vi "SetExtSignalPol.vi"(8 "错误输入（无错误）":errorcluster, 10 "外同步信号极性":u8) -> (0 "错误输出":errorcluster)   [LabVIEW 2018]
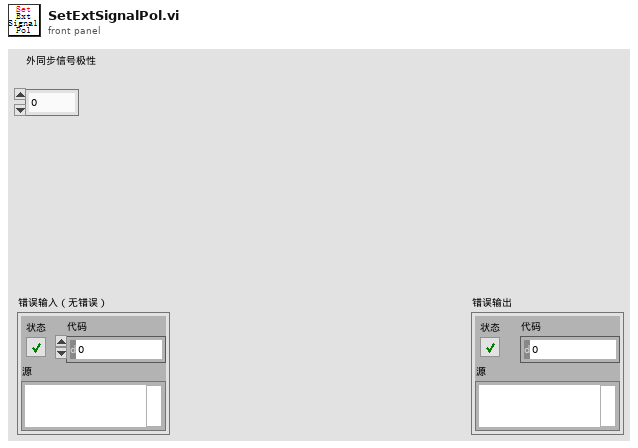
[diagram p1: front panel]
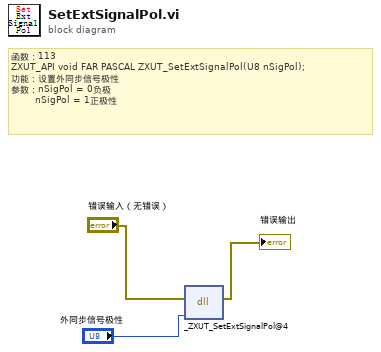
[diagram p0: block diagram]
diagram:
  # "函数：113\nZXUT_API void\tFAR PASCAL ZXUT_SetExtSignalPol(U8 nSigPol);\n功能：设置外同步信号极性\n参数：nSigPol = 0负极\n        nSigPol = 1正极性"
  n1 = dll-call lib="PTH2Rabs E软件项目超声超声子VI函数VI\tTCG处理ZXUTConfigMgr.dll" fn="_ZXUT_SetExtSignalPol@4"(error in="错误输入（无错误）", "nSigPol"="外同步信号极性") -> (error out=→"错误输出":errorcluster)  [unwired: 4 in, 1 out]
